vi "PolyGegenbauer.vi"(1 "alpha":dbl, 2 "n":i32) -> (0 "Cna":dbl[](array[numeric]))   [LabVIEW 2018, in "NI_AALPro.lvlib"]
uses:
  <vilib>/Analysis/NI_AALPro.lvlib
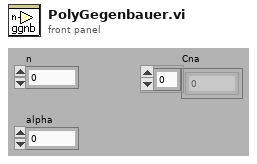
[diagram p1: front panel]
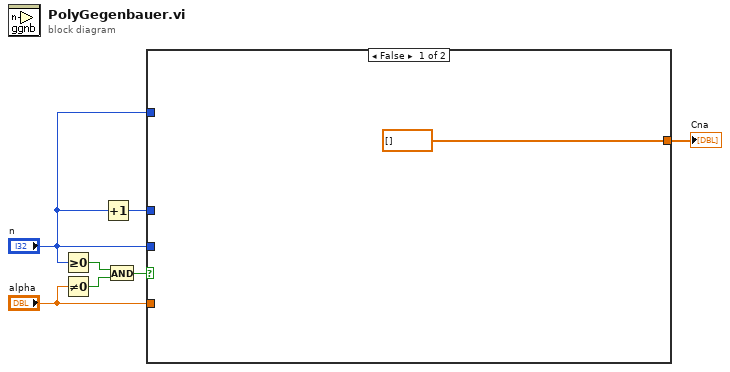
[diagram p0: block diagram]
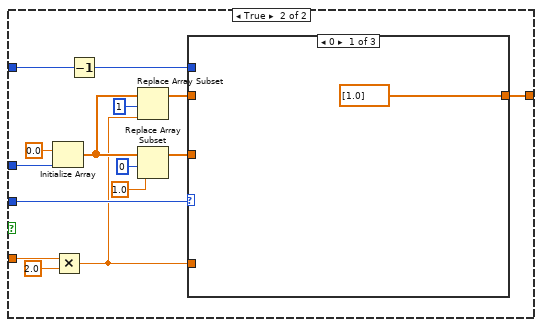
[diagram p2: hidden frame]
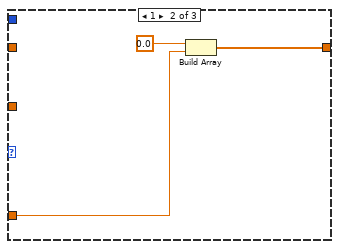
[diagram p3: hidden frame]
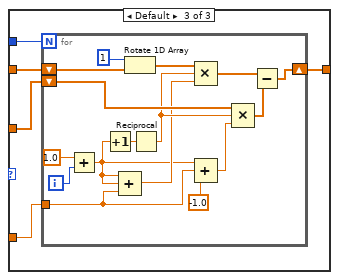
[diagram p4: hidden frame]
diagram:
  n1 = Greater Or Equal To 0?(x="n") -> (x >= 0?=w3:bool)
  n2 = Not Equal To 0?(x="alpha") -> (x != 0?=w2:bool)
  n3 = Increment(x="n") -> (x+1=w7:i32)
  n4 = And(x=w3, y=w2) -> (x .and. y?=w1:bool)
  n5 = case shown="False" w1 {
    tunnel: "n" -> [_ w23]
    tunnel: w7 -> [_ w16]
    tunnel: "n" -> [_ w14]
    tunnel: [dbl[] [] ("Tn(x)") w15] -> w5
    tunnel: "alpha" -> [_ w12]
    frame False {
    }
    frame True {
      n6 = Initialize Array(0.0 ("element"), w16) -> (w20:dbl[])
      n7 = Multiply(x=w12, y=2.0) -> (x*y=w10:dbl)
      n8 = Decrement(x=w14) -> (x-1=w13:i32)
      n9 = Replace Array Subset(array=w20, new element=w10, index=1) -> (w18:dbl[])
      n10 = Replace Array Subset(array=w20, new element=1.0 ("index"), index=0) -> (w17:dbl[])
      n11 = case shown="0" w23 {
        tunnel: w18 -> [_ _ w29]
        tunnel: w17 -> [_ _ w28]
        tunnel: w13 -> [_ _ w32]
        tunnel: [dbl[] [1.0] ("Tn(x)") w26 w31] -> w15
        tunnel: w10 -> [_ w25 w30]
        frame 0 {
        }
        frame 1 {
          n12 = Build Array(0.0, w25) -> (w26:dbl[])
        }
        frame Default {
          n13 = for {
            N: w32 -> [_]
            shift-right: [w42] -> w31
            shift-left: w29 -> [w38]
            shift-left: w28 -> [w47]
            tunnel: w30 -> [w40]
            i -> [w34]
            n14 = Add(x=1.0 ("index"), y=w34) -> (x+y=w35:dbl)
            n15 = Increment(x=w35) -> (x+1=w48:dbl)
            n16 = Compound Arithmetic op=ADD(w35, w35, w40) -> (w41:dbl)
            n17 = Rotate 1D Array(1:w38, 2:1 ("n")) -> (0:w37:dbl[])
            n18 = Reciprocal(x=w48) -> (1/x=w46:dbl)
            n19 = Compound Arithmetic op=MULTIPLY(w37, w46, w41) -> (w44:dbl[])
            n20 = Compound Arithmetic op=ADD(w35, w40, -1.0) -> (w45:dbl)
            n21 = Compound Arithmetic op=MULTIPLY(w47, w46, w45) -> (w43:dbl[])
            n22 = Subtract(x=w44, y=w43) -> (x-y=w42:dbl[])
          }
        }
      }
    }
  }
  "Cna" <- w5
